vi "Digital - Continuous Output.vi"() -> ()   [LabVIEW 2015]
doc: "This example demonstrates how to continuously re-generate digital output data. That output is hardware timed, so each sample is output on the next tick of the sample clock.\n\nSome hardware (e.g. M Series DAQ) must use an external sample clock for digital tasks. To view a complete list of available sample clock sources, consult the Device Routes table in Measurement and Automation Explorer.\n\nFor instructions on how to connect your signals to the DAQ device, refer to your device documentation."
uses:
  <vilib>/Utility/error.llb/DialogType.ctl
  <vilib>/DAQmx/write.llb/DAQmx Write (Analog 1D DBL 1Chan NSamp).vi
  <vilib>/DAQmx/write.llb/DAQmx Write (Digital 1D U32 1Chan NSamp).vi
  <vilib>/DAQmx/create/channels.llb/DAQmx Create Channel (DO-Digital Output).vi
  <vilib>/DAQmx/configure/timing.llb/DAQmx Timing (Sample Clock).vi
  <vilib>/DAQmx/configure/trigger.llb/DAQmx Start Trigger (Digital Edge).vi
  <vilib>/DAQmx/miscellaneous.llb/DAQmx Fill In Error Info.vi
  <vilib>/DAQmx/create/channels.llb/DAQmx Create Channel (AO-Voltage-Basic).vi
  <resource>/objmgr/daqmx.rc
panel:
  in  "Line(s)":tag="Dev1/port0/line0:7"
  in  "Stop":bool
  in  "Output Array":u32[](array[numeric])=[1, 2, 4, 8, 16, 32, 64, 128]
  in  "Trigger Type":enum32{"No Trigger", "Digital Start"}(tab)
  in  "Edge":i32(ring)=10280 items=["Rising"=10280, "Falling"=10171]
  in  "Digital Trigger Source":tag="PFI1"
  in  "Number of Samples":i32=1000
  in  "Sample Rate":dbl=1000.0
  in  "Sample Clock Source":tag="PFI0"
  out "Actual Sample Rate":dbl=1000.0 format="%0.2f"
  # "Channel Settings"
  # "Data to Write"
  # "Timing and Buffer Settings"
  # "Trigger Settings"
  # "To configure and use a start trigger you must have the necessary tab selected above.  Not all hardware supports triggering--refer to your device documentation for more info."
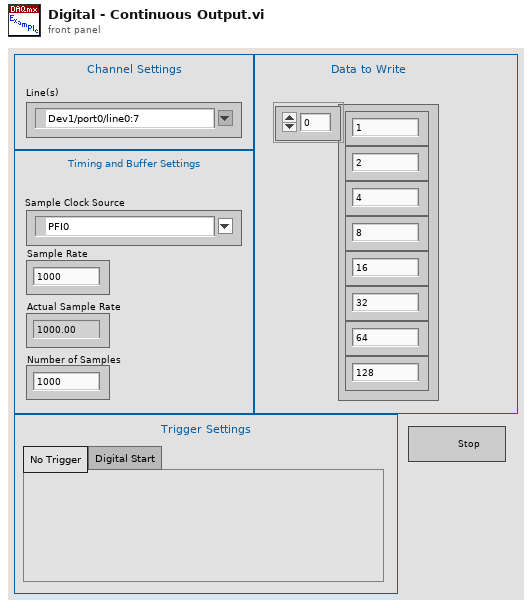
[diagram p1: front panel]
types:
  T1 = typedef "DialogType.ctl" = u16
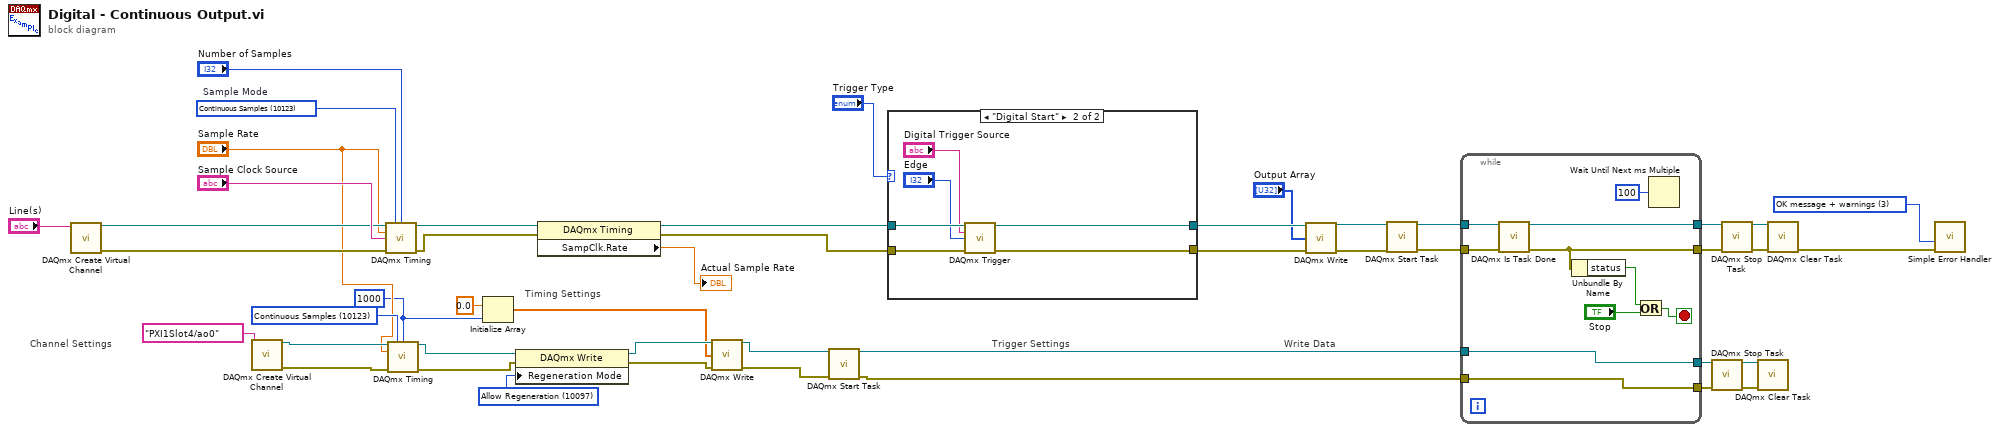
[diagram p0: block diagram]
diagram:
  w11 = 1000 ("samples per channel")
  w17 = 10097 items=["Allow Regeneration"=10097, "Do Not Allow Regeneration"=10158] ("RegenMode")
  w18 = 10123 items=["Finite Samples"=10178, "Continuous Samples"=10123, "Hardware Timed Single Point"=12522] ("sample mode")
  w22 = T1 3 items=["no dialog", "OK message", "continue or stop message", "OK message + warnings", "continue/stop + warnings"] ("type of dialog (OK msg:1)")
  w40 = 10123 items=["Finite Samples"=10178, "Continuous Samples"=10123, "Hardware Timed Single Point"=12522]  # Sample Mode
  # "Trigger Settings"
  # "Timing Settings"
  # "Write Data"
  # "Channel Settings"
  n1 = call-poly <vilib>:"DAQmx Create Virtual Channel.vi"("lines"="Line(s)") -> ("task out"=w43:refnum<k21>, "error out"=w42:errorcluster)  [unwired: 13 in]
  n2 = call-poly <vilib>:"DAQmx Create Virtual Channel.vi"("physical channels"=tag "PXI1Slot4/ao0") -> ("task out"=w20:refnum<k21>, "error out"=w19:errorcluster)  [unwired: 13 in]
  n3 = call-poly <vilib>:"DAQmx Timing.vi"("task/channels in"=w43, "sample mode"=w40, "samples per channel"="Number of Samples", "rate"="Sample Rate", "source"="Sample Clock Source", "error in"=w42) -> ("task out"=w39:refnum<k21>, "error out"=w38:errorcluster)  [unwired: 8 in]
  n4 = call-poly <vilib>:"DAQmx Timing.vi"("task/channels in"=w20, "sample mode"=w18, "samples per channel"=w11, "rate"="Sample Rate", "error in"=w19) -> ("task out"=w16:refnum<k21>, "error out"=w15:errorcluster)  [unwired: 9 in]
  n5 = Initialize Array(0.0 ("element"), w11) -> (w9:dbl[])
  n6 = property class="DAQmx Write"(reference=w16, error in=w15, "Regeneration Mode"=w17) -> (reference out=w13:refnum<k21>, error out=w12:errorcluster)
  n7 = property class="DAQmx Timing"(reference=w39, error in=w38) -> (reference out=w36:refnum<k21>, error out=w35:errorcluster, "SampClk.Rate"=→"Actual Sample Rate":dbl)
  n8 = call-poly <vilib>:"DAQmx Write.vi"("task/channels in"=w13, "data"=w9, "error in"=w12) -> ("task out"=w8:refnum<k21>, "error out"=w7:errorcluster)  [unwired: 10 in, 1 out]
  n9 = call <vilib>:"DAQmx Start Task.vi"("task/channels in"=w8, "error in"=w7) -> ("task out"=w3:refnum<k21>, "error out"=w1:errorcluster)  [unwired: 12 in]
  n10 = case shown="\"Digital Start\"" "Trigger Type" {
    tunnel: w36 -> [w48 w54]
    tunnel: w35 -> [w47 w53]
    tunnel: [w48 w52] -> w34
    tunnel: [w47 w51] -> w33
    frame "No Trigger", Default {
    }
    frame "Digital Start" {
      n11 = call-poly <vilib>:"DAQmx Trigger.vi"("task/channels in"=w54, "source"="Digital Trigger Source", "edge"="Edge", "error in"=w53) -> ("task out"=w52:refnum<k21>, "error out"=w51:errorcluster)  [unwired: 10 in]
    }
  }
  n12 = call-poly <vilib>:"DAQmx Write.vi"("task/channels in"=w34, "data"="Output Array", "error in"=w33) -> ("task out"=w31:refnum<k21>, "error out"=w30:errorcluster)  [unwired: 10 in, 1 out]
  n13 = call <vilib>:"DAQmx Start Task.vi"("task/channels in"=w31, "error in"=w30) -> ("task out"=w29:refnum<k21>, "error out"=w28:errorcluster)  [unwired: 12 in]
  n14 = while {
    tunnel: w29 -> [w64]
    tunnel: w28 -> [w63]
    tunnel: [w60] -> w23
    tunnel: [w62] -> w24
    tunnel: [w56] -> w4
    tunnel: w3 -> [w56]
    tunnel: [w55] -> w2
    tunnel: w1 -> [w55]
    stop <- w57 stop-if-true
    n15 = call <vilib>:"DAQmx Is Task Done.vi"("task/channels in"=w64, "error in"=w63) -> ("task out"=w62:refnum<k21>, "error out"=w60:errorcluster)  [unwired: 11 in, 1 out]
    n16 = Unbundle By Name(w60) -> ("status"=w59:bool)
    n17 = Or(x=w59, y="Stop") -> (x .or. y?=w57:bool)
    n18 = Wait Until Next ms Multiple(millisecond multiple=u32 100) -> ()  [unwired: 1 out]
  }
  n19 = call <vilib>:"DAQmx Stop Task.vi"("task/channels in"=w4, "error in"=w2) -> ("task out"=w6:refnum<k21>, "error out"=w5:errorcluster)  [unwired: 12 in]
  n20 = call <vilib>:"DAQmx Stop Task.vi"("task/channels in"=w24, "error in"=w23) -> ("task out"=w26:refnum<k21>, "error out"=w25:errorcluster)  [unwired: 12 in]
  n21 = call <vilib>:"DAQmx Clear Task.vi"("task in"=w6, "error in"=w5) -> ()  [unwired: 13 in, 1 out]
  n22 = call <vilib>:"DAQmx Clear Task.vi"("task in"=w26, "error in"=w25) -> ("error out"=w46:errorcluster)  [unwired: 13 in]
  n23 = call <vilib>:"Simple Error Handler.vi"("type of dialog (OK msg:1)"=w22, "error in (no error)"=w46) -> ()  [unwired: 3 in, 5 out]
